vi "Display Name.vi"(8 "error in (no error)":errorcluster, 11 "Name In":string) -> (0 "error out":errorcluster)   [LabVIEW 2018]
panel:
  out "String":string
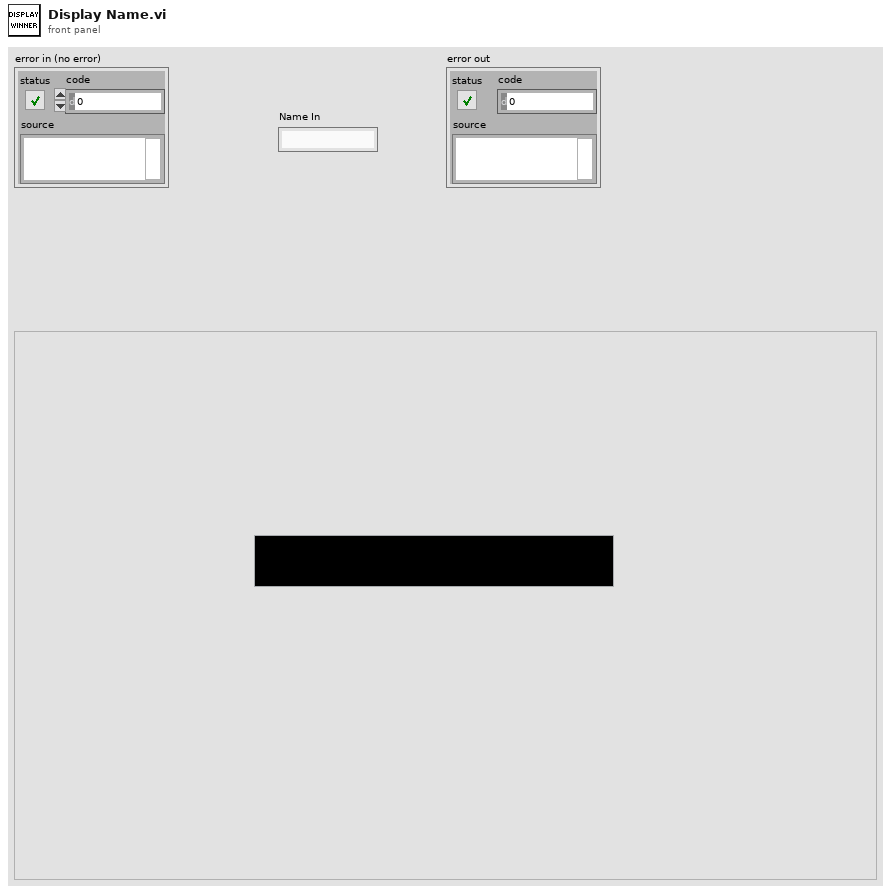
[diagram p1: front panel]
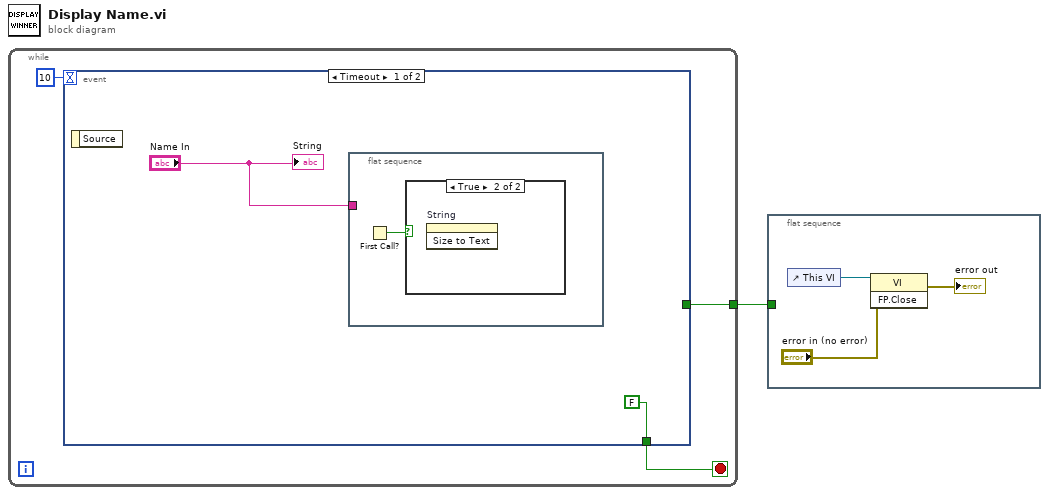
[diagram p0: block diagram]
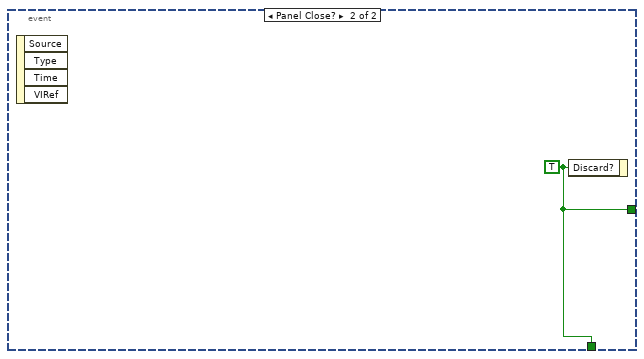
[diagram p3: hidden frame]
diagram:
  n1 = while {
    tunnel: [w2] -> w1
    stop <- w3 stop-if-true
    n2 = event shown="[0] Timeout" {
      selector: _ -> [_ _]
      dyn-events: _ -> [_ _]
      timeout: 10 -> [_ _]
      tunnel: [FALSE w8] -> w3
      tunnel: [_ w8] -> w2
      event Timeout {
        n3 = event-data() -> ()  [unwired: 1 in, 1 out]
        n4 = flat-sequence {
          tunnel: "Name In" -> [_]
          frame #0 {
            n5 = First Call?() -> (First Call?: T/F=w7:bool)
            n6 = case shown="True" w7 {
              frame False {
              }
              frame True {
                n7 = invoke on="String" class="Str" method="Size to Text"() -> ()  [unwired: 3 in, 3 out]
              }
            }
          }
        }
        "String" <- "Name In"
      }
      event Panel Close? {
        w8 = TRUE ("Discard?")
        n8 = event-data() -> ()  [unwired: 1 in, 4 out]
        n9 = event-data("Discard?"=w8) -> ()  [unwired: 1 in, 1 out]
      }
    }
  }
  n10 = flat-sequence {
    tunnel: w1 -> [_]
    frame #0 {
      n11 = control-ref of="This VI"() -> (w11:refnum<vi>)
      n12 = invoke class="VI" method="FP.Close"(reference=w11, error in="error in (no error)") -> (error out=→"error out":errorcluster)  [unwired: 1 in, 2 out]
    }
  }
